vi "STOP.vi"(8 "entrée d'erreur (pas d'erreur)":errorcluster, 11 "UV-VIS en entrée":refnum<class "UV-VIS.lvclass">) -> (0 "sortie d'erreur":errorcluster, 3 "UV-VIS en sortie":refnum<class "UV-VIS.lvclass">)   [LabVIEW 2015]
uses:
  UV-VIS.lvclass
  Detector.lvclass/Detector.ctl
  Detector.lvclass
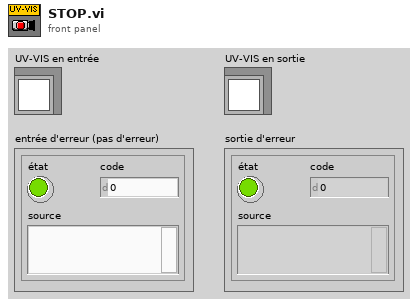
[diagram p1: front panel]
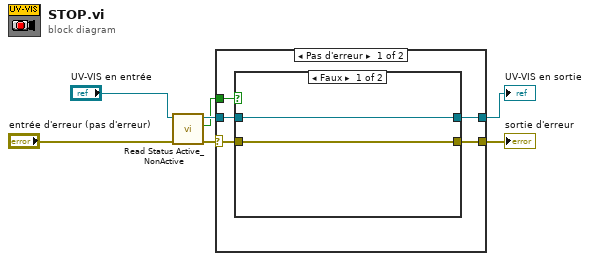
[diagram p0: block diagram]
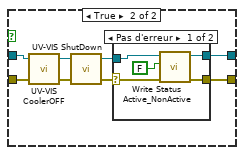
[diagram p2: hidden frame]
diagram:
  n1 = call "Read Status Active_NonActive.vi"("error in (no error)"="entrée d'erreur (pas d'erreur)", "Detector in"="UV-VIS en entrée") -> ("error out"=w3:errorcluster, "Status Active/NonActive"=w1:bool, "Detector out"=w2:refnum<class "UV-VIS.lvclass">)  [unwired: 7 in]
  n2 = case shown="Pas d'erreur" w3 {
    selector: w3 -> [w8 w31]
    tunnel: [w12 w31] -> w7
    tunnel: [w11 w30] -> w6
    tunnel: w2 -> [w10 w30]
    tunnel: w1 -> [w9 _]
    frame No Error {
      n3 = case shown="Faux" w9 {
        tunnel: [w13 w22] -> w12
        tunnel: [w14 w20] -> w11
        tunnel: w10 -> [w14 w16]
        tunnel: w8 -> [w13 w15]
        frame False {
        }
        frame True {
          n4 = call "UV-VIS CoolerOFF.vi"("error in (no error)"=w15, "UV-VIS  in"=w16) -> ("error out"=w17:errorcluster, "UV-VIS  out"=w18:refnum<class "UV-VIS.lvclass">)  [unwired: 1 in, 1 out]
          n5 = call "UV-VIS ShutDown.vi"("error in (no error)"=w17, "UV-VIS  in"=w18) -> ("error out"=w19:errorcluster, "UV-VIS  out"=w21:refnum<class "UV-VIS.lvclass">)  [unwired: 1 in, 1 out]
          n6 = case shown="Pas d'erreur" w19 {
            selector: w19 -> [w26 w28]
            tunnel: [w23 w29] -> w20
            tunnel: w21 -> [w27 w29]
            tunnel: [w25 w28] -> w22
            frame No Error {
              n7 = call "Write Status Active_NonActive.vi"("error in (no error)"=w26, "Status Active/NonActive"=FALSE, "Detector in"=w27) -> ("error out"=w25:errorcluster, "Detector out"=w23:refnum<class "UV-VIS.lvclass">)  [unwired: 7 in]
            }
            frame Error {
            }
          }
        }
      }
    }
    frame Error {
    }
  }
  "sortie d'erreur" <- w7
  "UV-VIS en sortie" <- w6
